vi "StopRecord.vi"(4 "error in (no error)":errorcluster, 6 "ClusterRefCtrlIN":T1, 7 "task/channels in":refnum<k21>) -> (0 "error out":errorcluster, 2 "RecStopped":bool, 3 "task out":refnum<k21>)   [LabVIEW 2017]
uses:
  <vilib>/DAQmx/write.llb/DAQmx Write (Digital Bool 1Line 1Point).vi
  DefDeType/ClusterRefCtrl.ctl
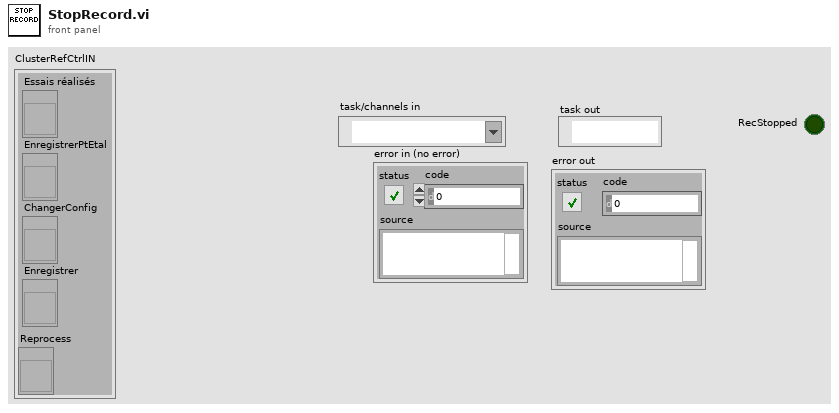
[diagram p1: front panel]
types:
  T1 = typedef "ClusterRefCtrl.ctl" = cluster{"Essais réalisés":refnum<vi>, "EnregistrerPtEtal":refnum<vi>, "ChangerConfig":refnum<vi>, "Enregistrer":refnum<vi>, "Reprocess":refnum<vi>}
  T2 = enum8{"Enabled", "Disabled", "Disabled and Grayed Out"}
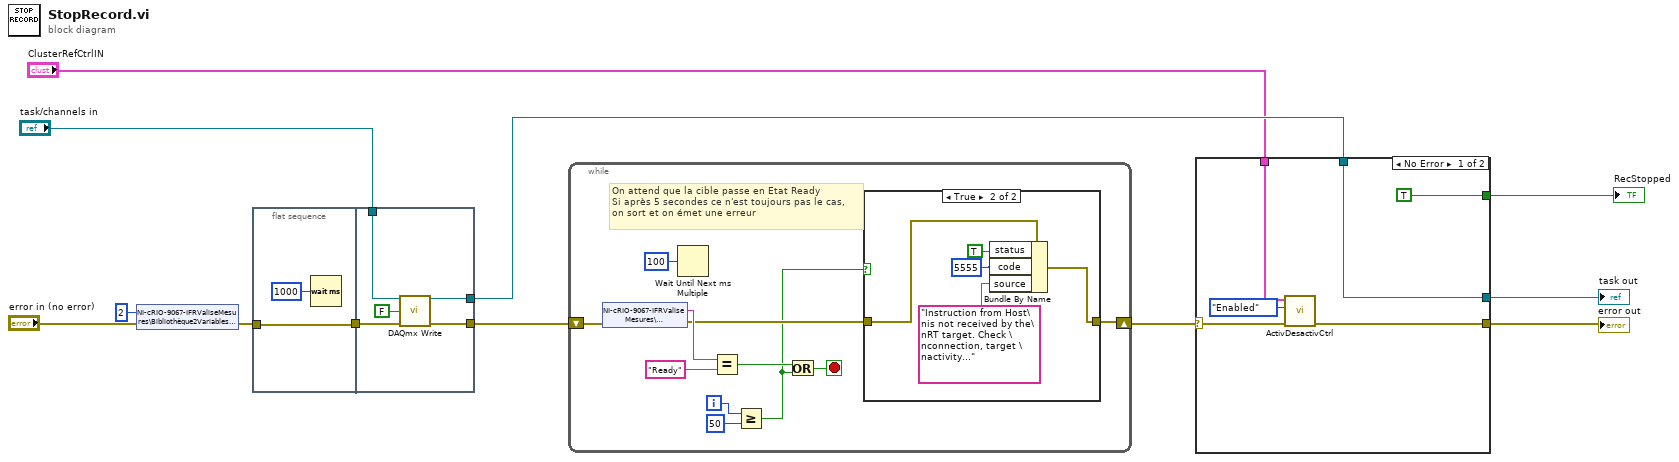
[diagram p0: block diagram]
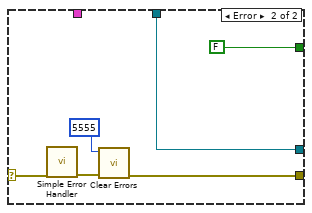
[diagram p2: hidden frame]
diagram:
  n1 = shared-variable "NI-cRIO-9067-IFRValiseMesures\\Bibliothèque2Variables.lvlib\\Instruction"(u8 2 ("Instruction"), error in="error in (no error)") -> (error out=w5:errorcluster)
  n2 = flat-sequence {
    tunnel: w5 -> [w13]
    tunnel: [w13] -> w6
    tunnel: w6 -> [w18]
    tunnel: "task/channels in" -> [w16]
    tunnel: [w17] -> w4
    tunnel: [w15] -> w2
    frame #0 {
      n3 = Wait (ms)(milliseconds to wait=u32 1000) -> ()  [unwired: 1 out]
    }
    frame #1 {
      n4 = call-poly <vilib>:"DAQmx Write.vi"("task/channels in"=w16, "data"=FALSE, "error in"=w18) -> ("task out"=w15:refnum<k21>, "error out"=w17:errorcluster)  [unwired: 10 in, 1 out]
    }
  }
  n5 = while {
    shift-right: [w20] -> w10
    shift-left: w4 -> [w30]
    i -> [w26]
    stop <- w23 stop-if-true
    # "On attend que la cible passe en Etat Ready\nSi après 5 secondes ce n'est toujours pas le cas, \non sort et on émet une erreur"
    n6 = shared-variable "NI-cRIO-9067-IFRValiseMesures\\Bibliothèque2Variables.lvlib\\RTState"(error in=w30) -> (w29:string, error out=w22:errorcluster)
    n7 = Wait Until Next ms Multiple(millisecond multiple=u32 100) -> ()  [unwired: 1 out]
    n8 = Equal?(x=w29, y="Ready") -> (x = y?=w24:bool)
    n9 = Greater Or Equal?(x=w26, y=50) -> (x >= y?=w21:bool)
    n10 = Or(x=w24, y=w21) -> (x .or. y?=w23:bool)
    n11 = case shown="True" w21 {
      tunnel: w22 -> [w31 w36]
      tunnel: [w31 w32] -> w20
      frame False {
      }
      frame True {
        n12 = Bundle By Name(cluster=w36, "status"=TRUE, "code"=5555, "source"="Instruction from Host\nis not received by the\nRT target. Check \nconnection, target \nactivity...") -> (w32:errorcluster)
      }
    }
  }
  n13 = case shown="No Error" w10 {
    selector: w10 -> [w40 w47]
    tunnel: w2 -> [w41 w48]
    tunnel: [w39 w44] -> w8
    tunnel: [w41 w48] -> w9
    tunnel: [TRUE ("RecStarted") FALSE ("RecStarted")] -> w7
    tunnel: "ClusterRefCtrlIN" -> [w37 _]
    frame No Error {
      n14 = call "ActivDesactivCtrl.vi"("error in (no error)"=w40, "Disabled"=T2."Enabled", "Cluster"=w37) -> ("error out"=w39:errorcluster)  [unwired: 4 in]
    }
    frame Error {
      n15 = call <vilib>:"Simple Error Handler.vi"("error in (no error)"=w47) -> ("error out"=w46:errorcluster)  [unwired: 4 in, 4 out]
      n16 = call <vilib>:"Clear Errors.vi"("error in (no error)"=w46, "specific error code to clear (0: all)"=5555) -> ("error out"=w44:errorcluster)  [unwired: 4 in, 1 out]
    }
  }
  "task out" <- w9
  "error out" <- w8
  "RecStopped" <- w7
